vi "SIM Registry LookupByTag.vi"(10 "Tag":string, 11 "Registry In":T1) -> (0 "Output Width":i32, 1 "Input Width":i32, 2 "Block Idx":i32, 3 "Registry Out":T1, 4 "Num Disc States":i32, 5 "Number of States":i32, 6 "Disc State Idx":i32, 7 "State Array Idx":i32, 8 "Discrete ID":i32)   [LabVIEW 2017]
uses:
  <vilib>/Simulation/Implementation/Shared/SIM Registry.llb/SIM Simulation Registry.ctl
  <vilib>/Simulation/Implementation/Shared/SIM Registry.llb/SIM Registry Node Header.ctl
  <vilib>/Simulation/Implementation/Shared/SIM Registry.llb/SIM Registry Node Record.ctl
  <vilib>/Simulation/Implementation/Shared/SIM trigger type.ctl
  <vilib>/Simulation/Implementation/Shared/SIM solver state data.ctl
  <vilib>/Simulation/Implementation/Shared/SIM limit type.ctl
  <vilib>/Simulation/Implementation/Shared/SIM discrete data.ctl
  <vilib>/Simulation/Implementation/Shared/SIM Discrete state data.ctl
  <vilib>/Simulation/Implementation/Shared/SIM Registry.llb/SIM Simulation Registry Error.ctl
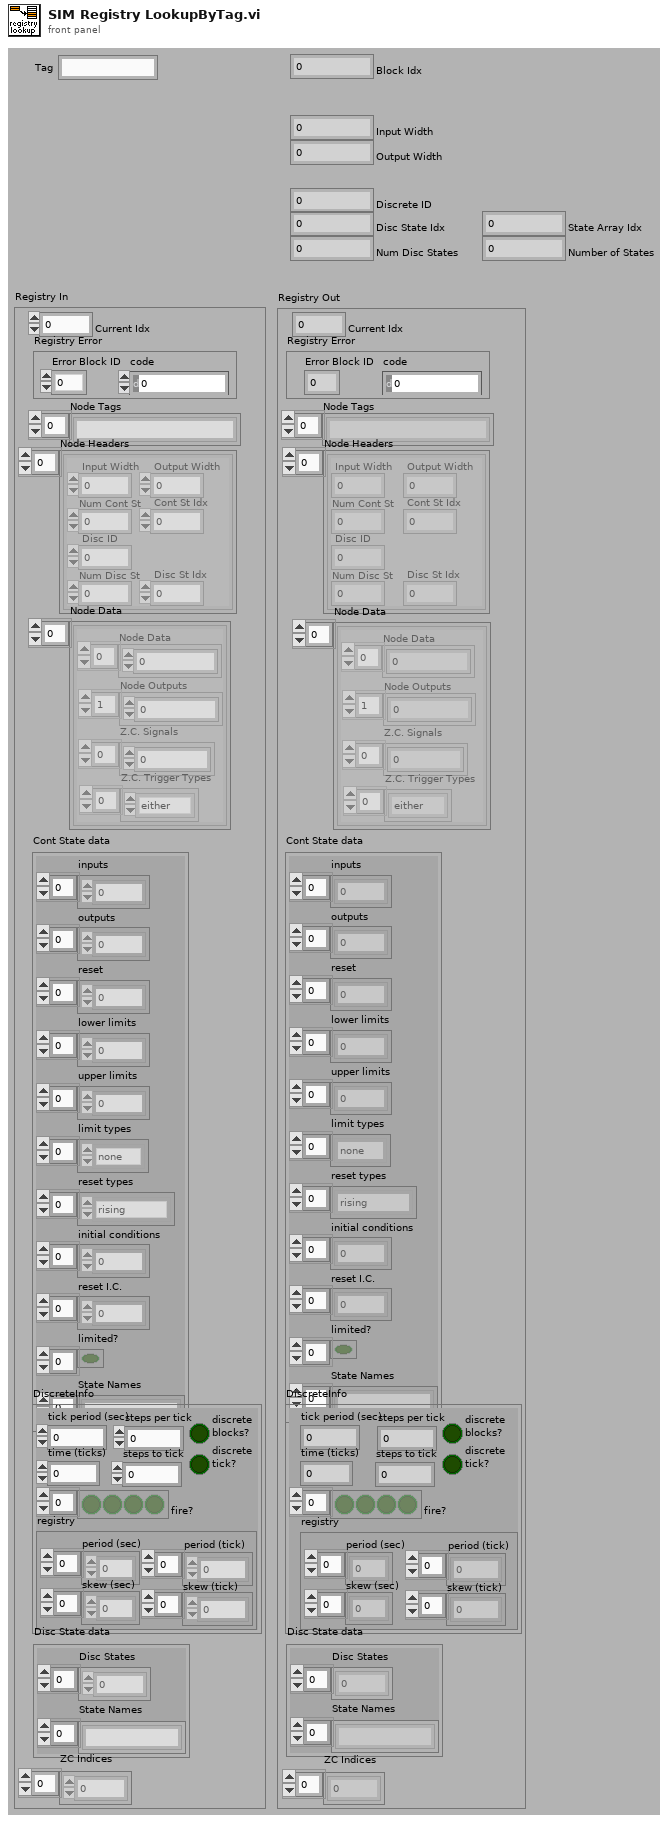
[diagram p1: front panel]
types:
  T1 = typedef "SIM Simulation Registry.ctl" = cluster{"Current Idx":i32, "Node Tags":string[], "Node Headers":T2[], "Node Data":T3[], "Cont State data":T5, "DiscreteInfo":T7, "Disc State data":T8, "Registry Error":T9, "ZC Indices":i32[]}
  T2 = typedef "SIM Registry Node Header.ctl" = cluster{"Input Width":i32, "Disc ID":i32, "Num Cont St":i32, "Cont St Idx":i32, "Num Disc St":i32, "Disc St Idx":i32, "Output Width":i32}
  T3 = typedef "SIM Registry Node Record.ctl" = cluster{"Node Data":dbl[], "Node Outputs":dbl[], "Z.C. Signals":dbl[], "Z.C. Trigger Types":T4[]}
  T4 = typedef "SIM trigger type.ctl" = enum16{"rising", "falling", "either", "none"}
  T5 = typedef "SIM solver state data.ctl" = cluster{"inputs":dbl[], "outputs":dbl[], "reset":dbl[], "lower limits":dbl[], "upper limits":dbl[], "limit types":T6[], "reset types":T4[], "initial conditions":dbl[], "reset I.C.":dbl[], "limited?":bool[], "State Names":string[]}
  T6 = typedef "SIM limit type.ctl" = enum16{"upper", "lower", "both", "none"}
  T7 = typedef "SIM discrete data.ctl" = cluster{"tick period (sec)":dbl, "time (ticks)":i32, "fire?":bool[], "registry":cluster{"period (sec)":dbl[], "skew (sec)":dbl[], "period (tick)":i32[], "skew (tick)":i32[]}, "discrete \nblocks?":bool, "steps per tick":dbl, "steps to tick":dbl, "discrete \ntick?":bool}
  T8 = typedef "SIM Discrete state data.ctl" = cluster{"Disc States":dbl[], "State Names":string[]}
  T9 = typedef "SIM Simulation Registry Error.ctl" = cluster{"Error Block ID":i32, "code":i32}
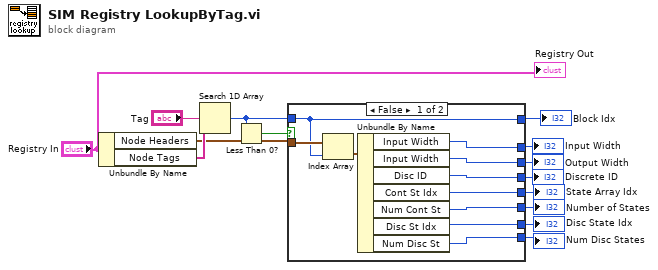
[diagram p0: block diagram]
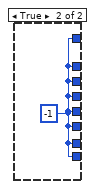
[diagram p2: hidden frame]
diagram:
  n1 = Unbundle By Name("Registry In") -> ("Node Headers"=w9:T2[], "Node Tags"=w14:string[])
  n2 = Search 1D Array(1D array=w14, element="Tag") -> (index of element=w7:i32)  [unwired: 1 out]
  n3 = Less Than 0?(x=w7) -> (x < 0?=w8:bool)
  n4 = case shown="False" w8 {
    tunnel: [w20 w25] -> w11
    tunnel: [w22 w25] -> w10
    tunnel: w9 -> [w24 _]
    tunnel: w7 -> [w20 _]
    tunnel: [w21 w25] -> w6
    tunnel: [w19 w25] -> w5
    tunnel: [w18 w25] -> w4
    tunnel: [w17 w25] -> w3
    tunnel: [w16 w25] -> w2
    tunnel: [w15 w25] -> w1
    frame False {
      n5 = Index Array(array=w24, index=w20) -> (element=w23:T2)
      n6 = Unbundle By Name(w23) -> ("Input Width"=w22:i32, "Input Width"=w15:i32, "Disc ID"=w21:i32, "Cont St Idx"=w19:i32, "Num Cont St"=w18:i32, "Disc St Idx"=w16:i32, "Num Disc St"=w17:i32)
    }
    frame True {
      w25 = -1 ("index of element")
    }
  }
  "Block Idx" <- w11
  "Input Width" <- w10
  "Discrete ID" <- w6
  "State Array Idx" <- w5
  "Number of States" <- w4
  "Disc State Idx" <- w2
  "Num Disc States" <- w3
  "Output Width" <- w1
  "Registry Out" <- "Registry In"
